vi "PCO_SetPseudoLut.vi"(8 "error in (no error)":errorcluster {"code" format="%x"}, 10 "pseudo_lut":u32[](array[numeric]), 11 "ph":u64) -> (0 "error out":errorcluster {"code" format="%x"}, 2 "ErrorMessage":i32 format="%x", 3 "ph out":u64)   [LabVIEW 2019, in "Convert.lvlib"]
doc: "int PCOCONVERT_API PCO_LoadPseudoLut(HANDLE ph, int format, char *filename);"
uses:
  Convert.lvlib
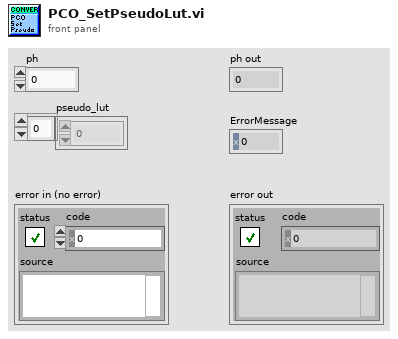
[diagram p1: front panel]
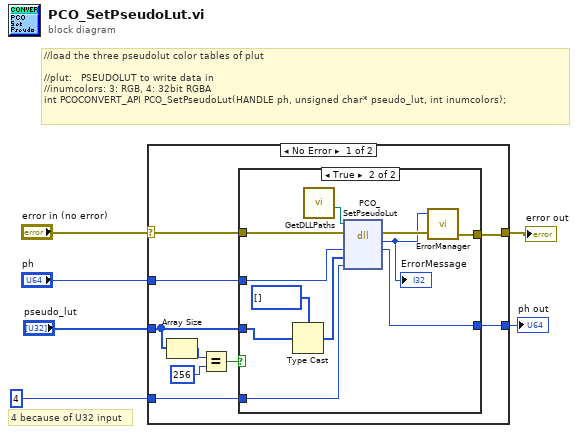
[diagram p0: block diagram]
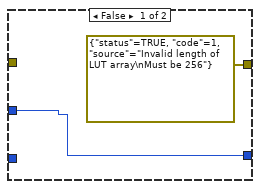
[diagram p2: hidden frame]
diagram:
  # "4 because of U32 input"
  # "//load the three pseudolut color tables of plut\n\n//plut:   PSEUDOLUT to write data in \n//inumcolors: 3: RGB, 4: 32bit RGBA\nint PCOCONVERT_API PCO_SetPseudoLut(HANDLE ph, unsigned char* pseudo_lut, int inumcolors);"
  n1 = case shown="No Error" "error in (no error)" {
    selector: "error in (no error)" -> [w11 w30]
    tunnel: "ph" -> [w15 w29]
    tunnel: [w14 w29] -> w5
    tunnel: "pseudo_lut" -> [w10 _]
    tunnel: 4 -> [w13 _]
    tunnel: [w12 w30] -> w4
    frame No Error {
      n2 = Array Size(array=w10) -> (size(s)=w9:i32)
      n3 = Equal?(x=w9, y=256) -> (x = y?=w7:bool)
      n4 = case shown="True" w7 {
        tunnel: w15 -> [w16 w28]
        tunnel: [w16 w27] -> w14
        tunnel: w13 -> [_ w26]
        tunnel: [errorcluster {"status"=TRUE, "code"=1, "source"="Invalid length of LUT array\nMust be 256"} ("error out") w24] -> w12
        tunnel: w11 -> [_ w22]
        tunnel: w10 -> [_ w19]
        frame False {
        }
        frame True {
          n5 = Type Cast(type=u8[] [] ("b32"), x=w19) -> (*(type *) &x=w18:u8[])
          n6 = call "GetDLLPaths.vi"() -> ("PCO_Conv_Path"=w21:path)  [unwired: 8 in, 3 out]
          n7 = dll-call lib="?" fn="PCO_SetPseudoLut"(path in=w21, error in=w22, "ph"=w28, "pseudo_lut"=w18, "inumcolors"=w26) -> (error out=w25:errorcluster, "return type"=w23:i32, "ph"=w27:u64)  [unwired: 3 in, 1 out]
          "ErrorMessage" <- w23
          n8 = call "ErrorManager.vi"("error in (no error)"=w25, "error code"=w23) -> ("error out"=w24:errorcluster)  [unwired: 2 in, 1 out]
        }
      }
    }
    frame Error {
    }
  }
  "ph out" <- w5
  "error out" <- w4
